vi "TW_ReadData.vi"(11 "Tag":T2) -> (2 "value":string)   [LabVIEW 2019]
uses:
  TW_Ctrl.ctl
panel:
  out "Comm":T1
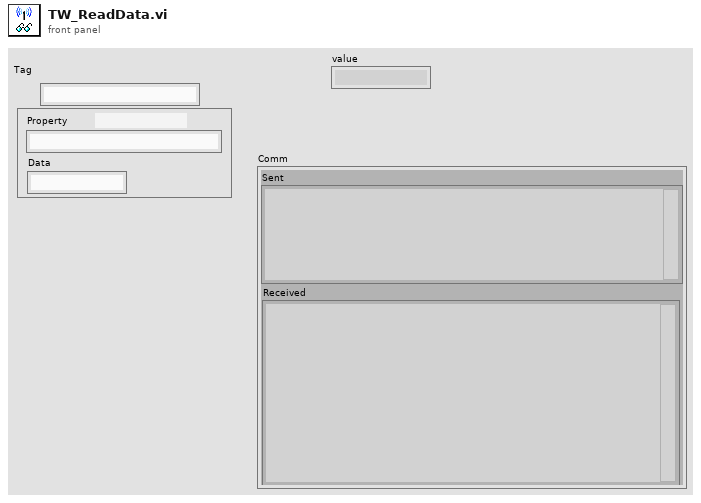
[diagram p1: front panel]
types:
  T1 = cluster{"url":string, "sent headers":string, "sent body":string, "headers":string, "body":string, "Sent":string, "Received":string}
  T2 = typedef "TW_Ctrl.ctl" = cluster{"Thing":string, "Property":string, "Type":string, "Data":string}
  T3 = enum16{"GET", "PUT", "POST", "MultiPOST", "DELETE"}
  T4 = cluster{"Name":string, "BaseURL":string, "AppKey":string, "Headers":string[], "Timeout":i32}
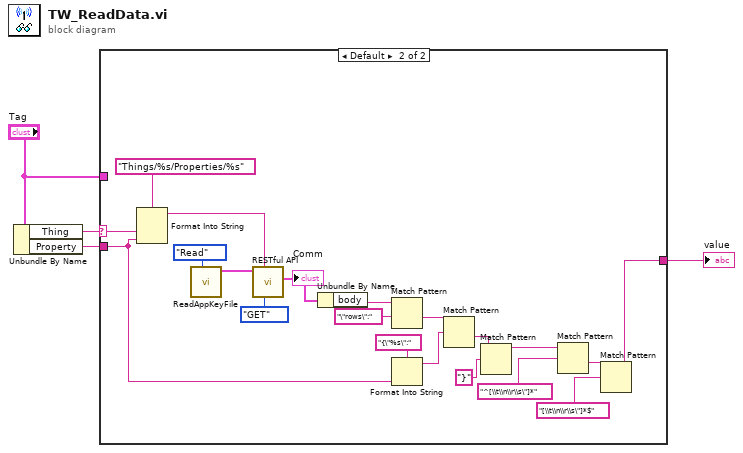
[diagram p0: block diagram]
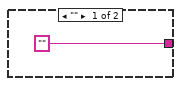
[diagram p2: hidden frame]
diagram:
  n1 = Unbundle By Name("Tag") -> ("Thing"=w4:string, "Property"=w2:string)
  n2 = case shown="Default" w4 {
    selector: w4 -> [_ w20]
    tunnel: "Tag" -> [_ _]
    tunnel: w2 -> [_ w17]
    tunnel: ["" ("body") w6] -> w1
    frame "" {
    }
    frame Default {
      n3 = Format Into String(format string="Things/%s/Properties/%s" ("url"), w20, w17) -> (resulting string=w25:string)  [unwired: 2 in, 1 out]
      n4 = call "ReadAppKeyFile.vi"("Task"=enum16{"Read", "Write"}."Read") -> ("Device Out"=w24:T4)  [unwired: 8 in, 2 out]
      n5 = call "RESTful API.vi"("Method"=T3."GET", "url"=w25, "Device In"=w24) -> ("Comm"=w19:T1)  [unwired: 6 in, 2 out]
      "Comm" <- w19
      n6 = Unbundle By Name(w19) -> ("body"=w14:string)
      n7 = Match Pattern(string=w14, regular expression="\"rows\":") -> (after substring=w13:string)  [unwired: 1 in, 3 out]
      n8 = Format Into String(format string="{\"%s\":" ("regular expression"), w17) -> (resulting string=w16:string)  [unwired: 2 in, 1 out]
      n9 = Match Pattern(string=w13, regular expression=w16) -> (after substring=w11:string)  [unwired: 1 in, 3 out]
      n10 = Match Pattern(string=w11, regular expression="}") -> (before substring=w9:string)  [unwired: 1 in, 3 out]
      n11 = Match Pattern(string=w9, regular expression="^[\\t\\n\\r\\s\"]*") -> (after substring=w7:string)  [unwired: 1 in, 3 out]
      n12 = Match Pattern(string=w7, regular expression="[\\t\\n\\r\\s\"]*$") -> (before substring=w6:string)  [unwired: 1 in, 3 out]
    }
  }
  "value" <- w1
